vi "mult_process_premade.vi"() -> ()   [LabVIEW 2013]
uses:
  results_cluster.ctl
panel:
  in  "Строка форматирования":string="%_5f ± %_3f; %_2f"
  out "Результат измерений":string
  in  "Pдов":dbl=0.95
  in  "Границы НСП":dbl
  out "Результаты обработки":T1 {"Dдов рез" format="%#.4g"; "S сумм" format="%#.4g"; "К" format="%#.4g"; "Dдов случ." format="%#.4g"; "Sхср" format="%#.4g"; "S" format="%#.4g"}
  in  "Записать результат":bool
  in  "Получить данные":bool
  in  "Вычислить Dдов":bool
  out "Ряд измерений":dbl[](graph)
  in  "Стоп":bool
  in  "Вычислить оценки":bool
  in  "Путь":path caption="Путь к файлу"
  # "Обработка результатов многократных измерений"
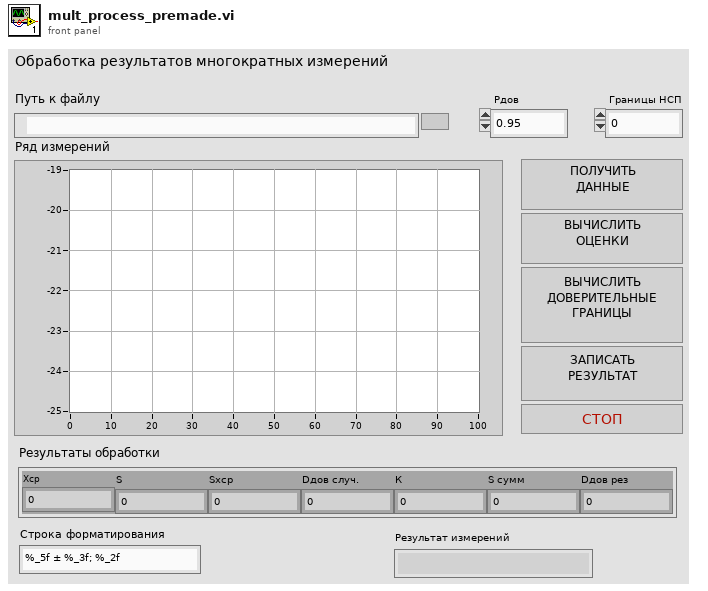
[diagram p1: front panel]
types:
  T1 = typedef "results_cluster.ctl" = cluster{"Xср":dbl, "S":dbl, "Sхср":dbl, "Dдов случ.":dbl, "К":dbl, "S сумм":dbl, "Dдов рез":dbl}
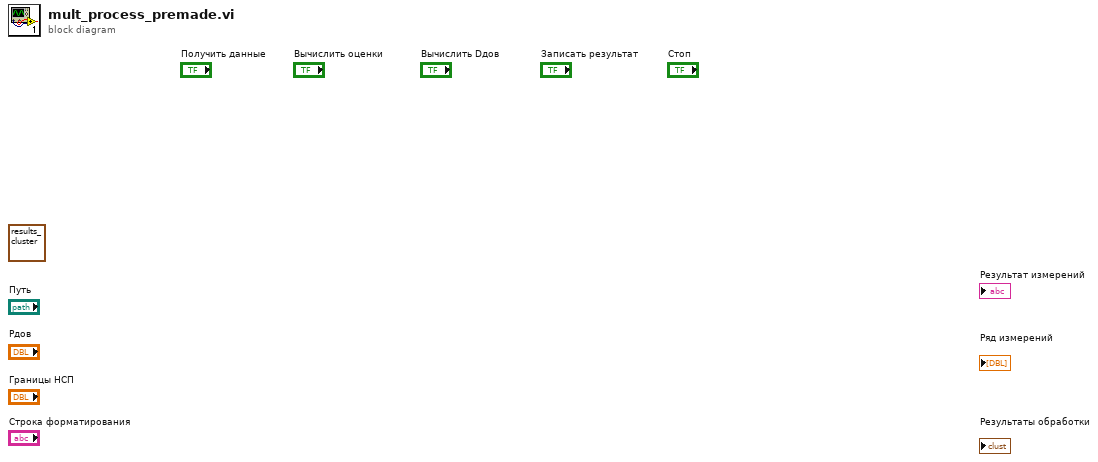
[diagram p0: block diagram]
diagram:
  (unwired) T1 {"Xср"=1.3199999999999998, "S"=0.130384048104053, "Sхср"=0.05830951894845301, "Dдов случ."=0.16189317847087023, "К"=2.43060784036949, "S сумм"=0.06506407098647712, "Dдов рез"=0.15814524106608838} ("Результаты обработки")
